vi "shell32_DragAcceptFiles.vi"(7 "Accept(T)":bool=TRUE, 8 "error in (no error)":errorcluster caption="错误输入（无错误）", 11 "hWnd":u32) -> (0 "error out":errorcluster caption="错误输出", 3 "dup hWnd":u32)   [LabVIEW 2011]
doc: "标识窗口是否接受从shell拖放过来的文件。"
uses:
  shell32.dll
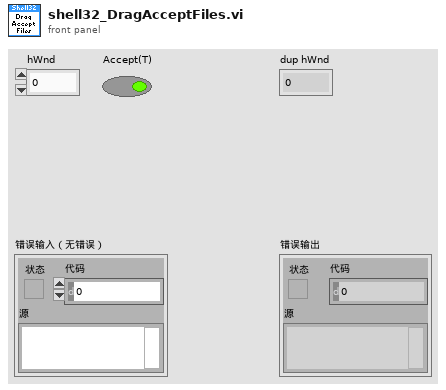
[diagram p1: front panel]
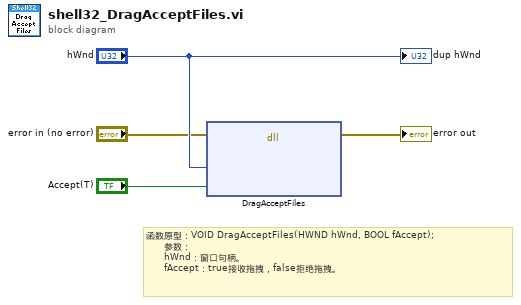
[diagram p0: block diagram]
diagram:
  # "函数原型：VOID DragAcceptFiles(HWND hWnd, BOOL fAccept);\n　　参数：\n　　hWnd：窗口句柄。\n　　fAccept：true接收拖拽，false拒绝拖拽。"
  n1 = dll-call lib="shell32.dll" fn="DragAcceptFiles"(error in="error in (no error)", "hWnd"="hWnd", "Accept"="Accept(T)") -> (error out=→"error out":errorcluster)  [unwired: 5 in, 1 out]
  "dup hWnd" <- "hWnd"
